vi "test_GetClusterElementsByName.vi"() -> ()   [LabVIEW 2013]
uses:
  source/TypeDescriptor/VariantToDescriptorElements.vi
  source/Conversions/String to Segments.vi
  source/Variant/OpenVariant.lvlib
panel:
  out "x = y? 2":bool
  out "x = y?":bool
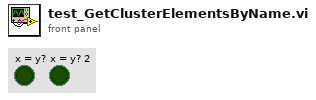
[diagram p1: front panel]
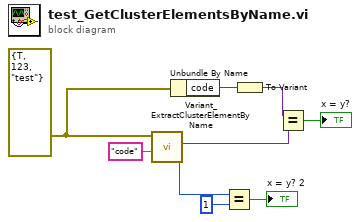
[diagram p0: block diagram]
diagram:
  w8 = errorcluster {"status"=TRUE, "code"=123, "source"="test"} ("error constant")
  n1 = call "Variant_ExtractClusterElementByName.vi"("name"="code", "Cluster"=w8) -> ("index"=w7:i32, "Element"=w4:variant)  [unwired: 7 in, 1 out]
  n2 = Unbundle By Name(w8) -> ("code"=w5:i32)
  n3 = Equal?(x=w7, y=1) -> (x = y?=→"x = y? 2":bool)
  n4 = To Variant(anything=w5) -> (Variant=w3:variant)
  n5 = Equal?(x=w3, y=w4) -> (x = y?=→"x = y?":bool)
